vi "HTTP-Parse Response Code.vi"(0 "headers":string) -> (4 "code":i32)   [LabVIEW 2020]
uses:
  <vilib>/regexp/Match Regular Expression.xnode
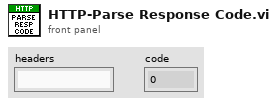
[diagram p1: front panel]
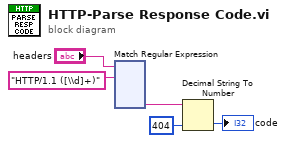
[diagram p0: block diagram]
diagram:
  n1 = xnode "Match Regular Expression"("input string"="headers", "regular expression"="HTTP/1.1 ([\\d]+)") -> ("submatch 1"=w3:string)  [unwired: 4 in, 5 out]
  n2 = Decimal String To Number(string=w3, default (0L)=404 ("default (0 I32)")) -> (number=→"code":i32)  [unwired: 1 in, 1 out]
